vi "PH_PPPA_PowerUnit.constructor.vi"(0 "name":string, 2 "data in":string, 5 "error in(no error)":errorcluster) -> (14 "i ref out":refnum<vi>, 16 "data out":string, 19 "error out":errorcluster)   [LabVIEW 2014, in "PH_PPPA_PowerUnit.lvlib"]
doc: "This class is forseen to control a PreAmp Power Unit. Actually it controls several device layer classes. The head itself is fully operational, but should be used via the PHELIX_Sequencer class only. It has an own state machine.\n\nThis class is part of the PHELIX application layer.\n\nauthor: Stefan Götte, GSI\n\nLicense Agreement for this software:\n\nCopyright (C)\nGesellschaft für Schwerionenforschung, GSI\nPlanckstr. 1\n64291 Darmstadt\nGermany\n\nContact: D.Beck@gsi.de \n\nThis program is free software; you can redistribute it and/or modify it under the terms of the \nGNU General Public License as published by the Free Software Foundation; either version 2 of \nthe license, or (at your option) any later version.\n\nThis program is distributed in the hope that it will be useful, but WITHOUT ANY WARRANTY; \nwithout even the implied warranty of MERCHANTABILITY or FITNESS FOR A PARTICULAR PURPOSE. See the GNU General License for more details (http://www.gnu.org).\n\nGesellschaft für Schwerionenforschung, GSI\nPlanckstr. 1, 64291 Darmstadt, Germany\nFor all questions and ideas contact: M.Richter@gsi.de, H.Brand@gsi.de or D.Beck@gsi.de.\nLast update: 16-JUN-2004"
uses:
  PH_PPPA_PowerUnit.lvlib
  PH_Basics/PH_PowerUnit_BaseClass/PH_PowerUnit_BaseClass.lvlib
  PH_Basics/PH_Class/PH_Class.lvlib
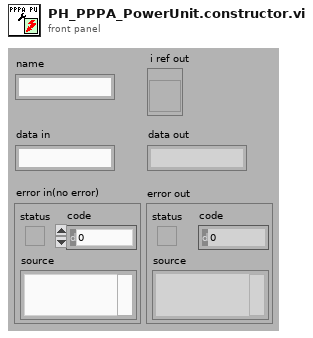
[diagram p1: front panel]
types:
  T1 = enum16{"SetAttribute", "GetAttribute", "CreateAttribute", "DestroyAttribute", "DestroyAllAtributes"}
  T2 = typedef "PH_PPPA_PowerUnit.lvlib/PH_PPPA_PowerUnit.i attribute.ctl" = cluster{"GUI Refs":cluster{"Ignitron":refnum<vi>, "Rossrelais":refnum<vi>, "Set Voltage":refnum<vi>, "PSU":refnum<vi>, "EOC":refnum<vi>, "Trigger":refnum<vi>}, "Ignitron":T3, "PSU":T5, "Dump Ross Relais":T6, "Trigger":cluster{"State Device":T4, "linked?":bool}, "Timing Settings":cluster{"Prdc Fast?":bool, "Default Value Periodic Interval":i32, "Mercury on since":dbl, "Warm up Time Mercury [s]":dbl}, "Set Voltage [V]":dbl, "19er Ignitionbox":string}
  T3 = typedef "PH_PP_Common.lvlib/PH_PP_Common.Ignitron Attributes.ctl" = cluster{"State Device":T4, "linked?":bool}
  T4 = typedef "PH_StatusHandler.lvlib/PH_StatusHandler.Status.ctl" = i16
  T5 = typedef "PH_PP_Common.lvlib/PH_PP_Common.PSU Attributes.ctl" = cluster{"lower limit [V]":dbl, "upper limit [V]":dbl, "Voltage set":bool, "State Device":T4, "linked?":bool}
  T6 = typedef "PH_PP_Common.lvlib/PH_PP_Common.Ross Relais Attributes.ctl" = cluster{"State Device":T4, "linked?":bool}
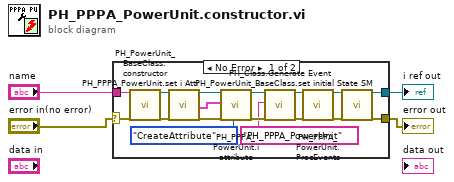
[diagram p0: block diagram]
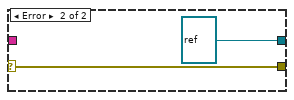
[diagram p2: hidden frame]
diagram:
  n1 = case shown="No Error" "error in(no error)" {
    selector: "error in(no error)" -> [w5 w23]
    tunnel: "name" -> [w13 _]
    tunnel: [w18 w23] -> w3
    tunnel: [w19 refnum<vi> refnum ("i ref out")] -> w2
    frame No Error {
      n2 = call "PH_PowerUnit_BaseClass.constructor.vi"("name"=w13, "error in(no error)"=w5) -> ("i ref out"=w6:refnum<vi>, "error out"=w7:errorcluster)  [unwired: 15 in, 1 out]
      n3 = call "PH_PPPA_PowerUnit.set i Attr.vi"("i ref in"=w6, "error in"=w7) -> ("i ref out"=w14:refnum<vi>, "i Attribute"=w16:T2, "error out"=w15:errorcluster)  [unwired: 15 in]
      n4 = call "PH_PPPA_PowerUnit.i attribute.vi"("VI Refnum"=w14, "CLASS.i attribute"=w16, "Action"=T1."CreateAttribute", "error in (no error)"=w15) -> ("VI Refnum out"=w12:refnum<vi>, "error out"=w11:errorcluster)  [unwired: 13 in, 1 out]
      n5 = call "PH_Class.Generate Event.vi"("i ref in"=w12, "Class"="PH_PPPA_PowerUnit", "error in (no error)"=w11) -> ("i ref out"=w10:refnum<vi>, "error out"=w9:errorcluster)  [unwired: 15 in]
      n6 = call "PH_PPPA_PowerUnit.ProcEvents.vi"("i ref in"=w10, "error in (no error)"=w9) -> ("i ref out"=w20:refnum<vi>, "error out"=w21:errorcluster)  [unwired: 16 in]
      n7 = call "PH_PowerUnit_BaseClass.set initial State SM.vi"("VI in"=w20, "error in (no error)"=w21) -> ("VI out"=w19:refnum<vi>, "error out"=w18:errorcluster)  [unwired: 16 in]
    }
    frame Error {
    }
  }
  "i ref out" <- w2
  "error out" <- w3
